vi "Bezahlen.vi"() -> ()   [LabVIEW 2023]
panel:
  out "Betrag erreicht":bool
  in  "Bezahlen":bool
  out "Restgeld":dbl
  in  "Storno":bool
  out "Guthaben":dbl
  in  "Preis":dbl
  in  "100 Euro":bool
  in  "50 Euro":bool
  in  "20 EUro":bool
  in  "10 Euro":bool
  in  "5 Euro":bool
  in  "2 Euro":bool
  in  "Stop Button":bool
  in  "1 Euro":bool
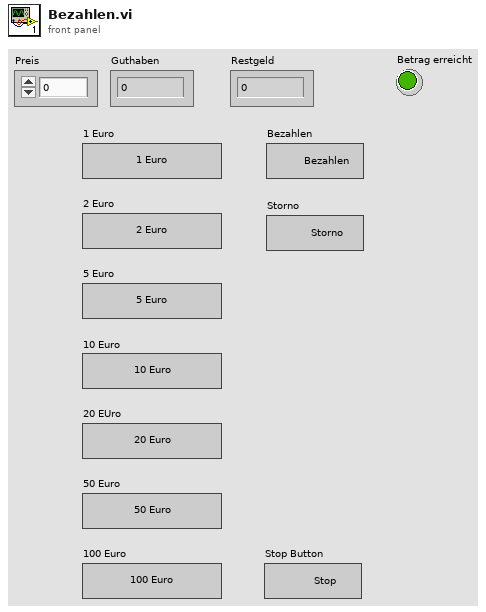
[diagram p1: front panel]
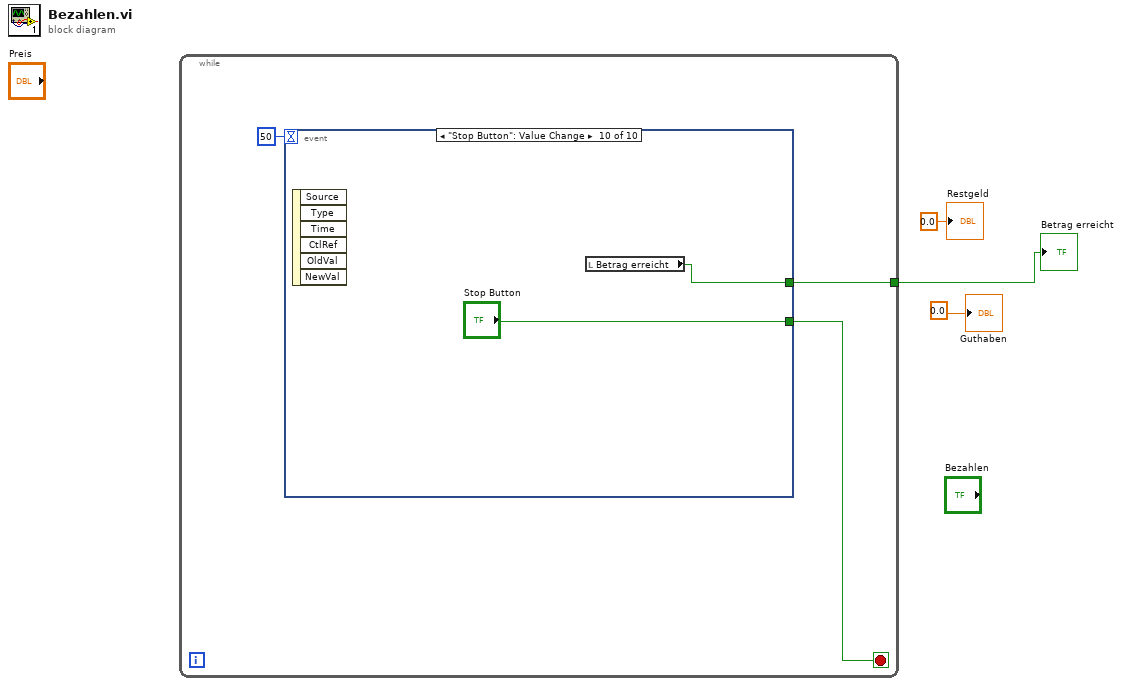
[diagram p0: block diagram]
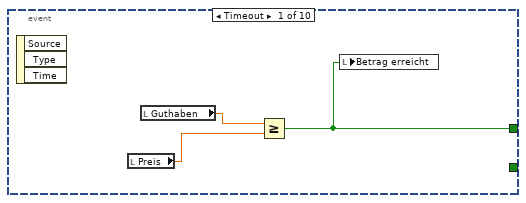
[diagram p2: hidden frame]
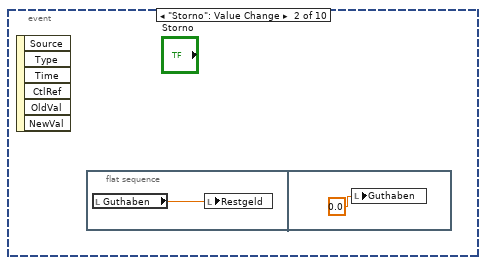
[diagram p3: hidden frame]
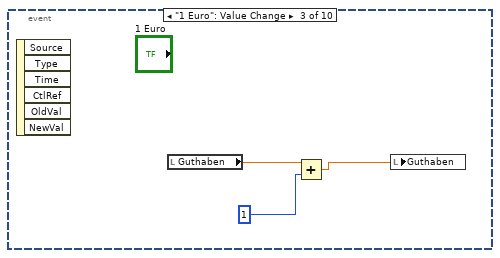
[diagram p4: hidden frame]
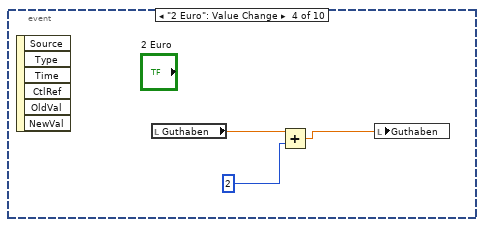
[diagram p5: hidden frame]
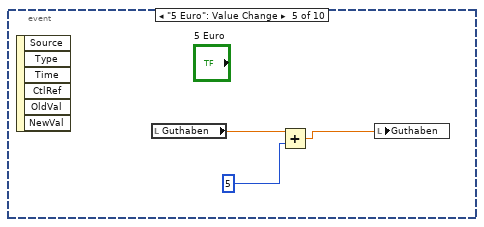
[diagram p6: hidden frame]
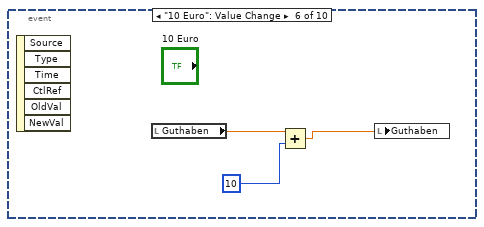
[diagram p7: hidden frame]
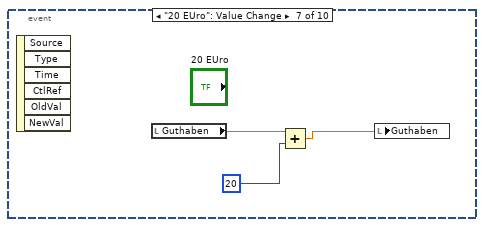
[diagram p8: hidden frame]
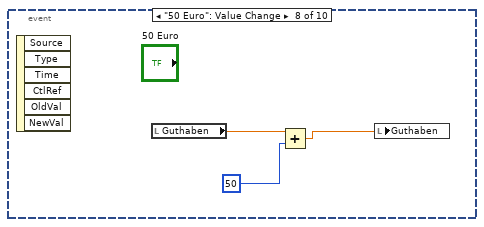
[diagram p9: hidden frame]
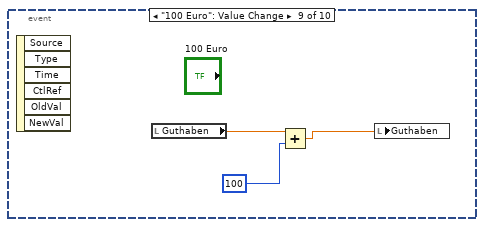
[diagram p10: hidden frame]
diagram:
  n1 = while {
    tunnel: [w4] -> w1
    stop <- w6 stop-if-true
    n2 = event shown="[9] \"Stop Button\": Value Change" {
      selector: _ -> [_ _ _ _ _ _ _ _ _ _]
      dyn-events: _ -> [_ _ _ _ _ _ _ _ _ _]
      timeout: 50 -> [_ _ _ _ _ _ _ _ _ _]
      tunnel: [_ _ _ _ _ _ _ _ _ "Stop Button"] -> w6
      tunnel: [w7 _ _ _ _ _ _ _ _ w33] -> w4
      event Timeout {
        n3 = event-data() -> ()  [unwired: 1 in, 3 out]
        n4 = local read "Preis"() -> (w8:dbl)
        n5 = local read "Guthaben"() -> (w9:dbl)
        n6 = Greater Or Equal?(x=w9, y=w8) -> (x >= y?=w7:bool)
        n7 = local write "Betrag erreicht"(w7) -> ()
      }
      event "Storno": Value Change {
        n8 = event-data() -> ()  [unwired: 1 in, 6 out]
        n9 = flat-sequence {
          frame #0 {
            n10 = local read "Guthaben"() -> (w10:dbl)
            n11 = local write "Restgeld"(w10) -> ()
          }
          frame #1 {
            n12 = local write "Guthaben"(0.0 ("Guthaben")) -> ()
          }
        }
      }
      event "1 Euro": Value Change {
        n13 = event-data() -> ()  [unwired: 1 in, 6 out]
        n14 = local read "Guthaben"() -> (w13:dbl)
        n15 = Add(x=w13, y=1) -> (x+y=w12:dbl)
        n16 = local write "Guthaben"(w12) -> ()
      }
      event "2 Euro": Value Change {
        n17 = event-data() -> ()  [unwired: 1 in, 6 out]
        n18 = local read "Guthaben"() -> (w16:dbl)
        n19 = Add(x=w16, y=2) -> (x+y=w15:dbl)
        n20 = local write "Guthaben"(w15) -> ()
      }
      event "5 Euro": Value Change {
        n21 = event-data() -> ()  [unwired: 1 in, 6 out]
        n22 = local read "Guthaben"() -> (w19:dbl)
        n23 = Add(x=w19, y=5) -> (x+y=w18:dbl)
        n24 = local write "Guthaben"(w18) -> ()
      }
      event "10 Euro": Value Change {
        n25 = event-data() -> ()  [unwired: 1 in, 6 out]
        n26 = local read "Guthaben"() -> (w22:dbl)
        n27 = Add(x=w22, y=10) -> (x+y=w21:dbl)
        n28 = local write "Guthaben"(w21) -> ()
      }
      event "20 EUro": Value Change {
        n29 = event-data() -> ()  [unwired: 1 in, 6 out]
        n30 = local read "Guthaben"() -> (w25:dbl)
        n31 = Add(x=w25, y=20) -> (x+y=w24:dbl)
        n32 = local write "Guthaben"(w24) -> ()
      }
      event "50 Euro": Value Change {
        n33 = event-data() -> ()  [unwired: 1 in, 6 out]
        n34 = local read "Guthaben"() -> (w28:dbl)
        n35 = Add(x=w28, y=50) -> (x+y=w27:dbl)
        n36 = local write "Guthaben"(w27) -> ()
      }
      event "100 Euro": Value Change {
        n37 = event-data() -> ()  [unwired: 1 in, 6 out]
        n38 = local read "Guthaben"() -> (w31:dbl)
        n39 = Add(x=w31, y=100) -> (x+y=w30:dbl)
        n40 = local write "Guthaben"(w30) -> ()
      }
      event "Stop Button": Value Change {
        n41 = event-data() -> ()  [unwired: 1 in, 6 out]
        n42 = local read "Betrag erreicht"() -> (w33:bool)
      }
    }
  }
  "Betrag erreicht" <- w1
  "Guthaben" <- 0.0 ("Preis")
  "Restgeld" <- 0.0 ("Restgeld")
